vi "Save Recall Instrument Settings.vi"(8 "error in (no error)":errorcluster, 9 "Memory Location (1)":u32=1, 10 "Operation (0: Recall)":i32(ring) items=["Recall", "Save"], 11 "VISA resource name":refnum<visa-resource-name>) -> (0 "error out":errorcluster, 3 "VISA resource name out":refnum<visa-resource-name>)   [LabVIEW 2023, in "Keithley DMM6500 DAQ6500 Series.lvlib"]
doc: "Save or recall instrument settings to different memory locations."
uses:
  <instrlib>/Keithley DMM6500 DAQ6500 Series/Keithley DMM6500 DAQ6500 Series.lvlib
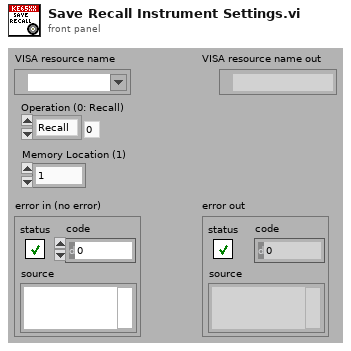
[diagram p1: front panel]
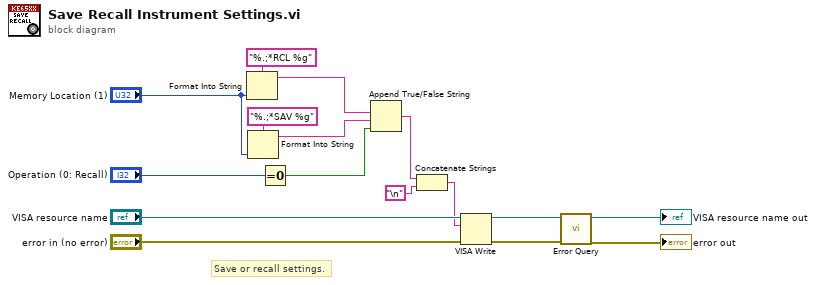
[diagram p0: block diagram]
diagram:
  # "Save or recall settings."
  n1 = Format Into String(format string="%.;*RCL %g", "Memory Location (1)") -> (resulting string=w2:string)  [unwired: 2 in, 1 out]
  n2 = Format Into String(format string="%.;*SAV %g", "Memory Location (1)") -> (resulting string=w3:string)  [unwired: 2 in, 1 out]
  n3 = Equal To 0?(x="Operation (0: Recall)") -> (x = 0?=w4:bool)
  n4 = Append True/False String(1:w4, 2:w3, 3:w2) -> (0:w1:string)  [unwired: 1 in]
  n5 = Concatenate Strings(w1, "\n") -> (w8:string)
  n6 = VISA Write(VISA resource name="VISA resource name", write buffer=w8, error in (no error)="error in (no error)") -> (VISA resource name out=w12:refnum<visa-resource-name>, error out=w11:errorcluster)  [unwired: 1 out]
  n7 = call <instrlib>:"Error Query.vi"("error in (no error)"=w11, "VISA resource name"=w12) -> ("error out"=→"error out":errorcluster, "VISA resource name out"=→"VISA resource name out":refnum<visa-resource-name>)  [unwired: 6 in, 2 out]
